vi "Trigger Plugin Discovery Internal.vi"(8 "error in (no error)":errorcluster, 10 "Trigger Discovery":T1, 11 "CIFPluginManager in":refnum<class "CIFPluginManager.lvclass">) -> (0 "error out":errorcluster)   [LabVIEW 2021, in "CIFPluginManager.lvclass"]
uses:
  CIFPluginManager.lvclass
  CIFPluginManager.lvclass/CIFPluginManager.ctl
  <vilib>/event_ctls.llb/usereventprio.ctl
  typedef/Discover Command.ctl
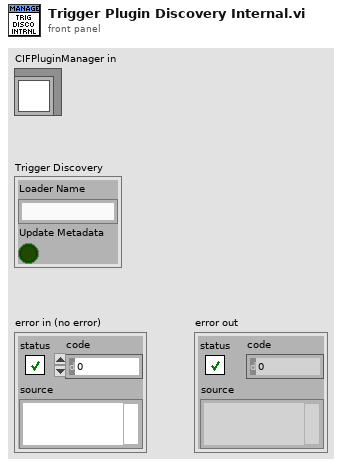
[diagram p1: front panel]
types:
  T1 = typedef "CIFPluginManager.lvclass/Discover Command.ctl" = cluster{"Loader Name":string, "Update Metadata":bool}
  T2 = typedef "usereventprio.ctl" = enum32{"high priority", "normal priority"}
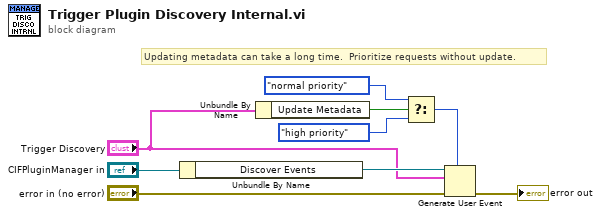
[diagram p0: block diagram]
diagram:
  # "Updating metadata can take a long time.  Prioritize requests without update."
  n1 = Unbundle By Name("CIFPluginManager in") -> ("Discover Events"=w6:refnum<user-event>)
  n2 = Unbundle By Name("Trigger Discovery") -> ("Update Metadata"=w4:bool)
  n3 = Select(t=usereventprio."normal priority" ("priority (normal)"), s=w4, f=usereventprio."high priority" ("priority (normal)")) -> (s? t:f=w1:T2)
  n4 = Generate User Event(priority (normal)=w1, user event=w6, event data cluster="Trigger Discovery", error in="error in (no error)") -> (error out=→"error out":errorcluster)  [unwired: 1 out]
